vi "Read FieldWidthY.vi"(0 "Field in":refnum<class "Field.lvclass">, 1 "error in (no error)":errorcluster) -> (2 "Field out":refnum<class "Field.lvclass">, 3 "FieldWidthY":i32=55, 4 "error out":errorcluster)   [LabVIEW 2014, in "Field.lvclass"]
uses:
  Field.lvclass
  Field.lvclass/Field.ctl
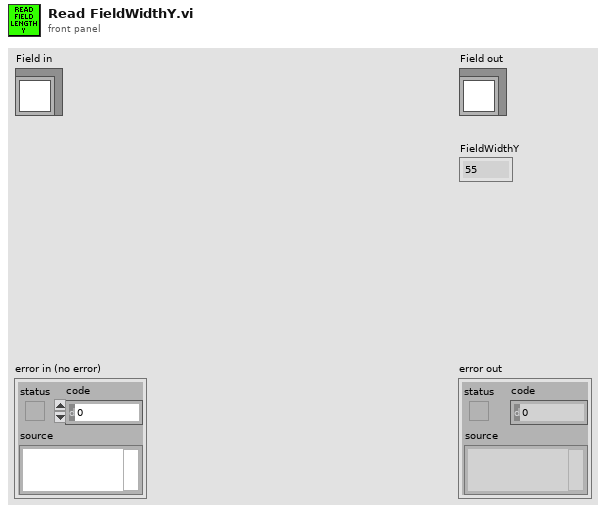
[diagram p1: front panel]
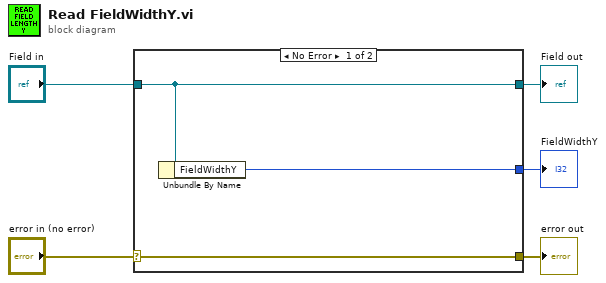
[diagram p0: block diagram]
diagram:
  n1 = case shown="No Error" "error in (no error)" {
    selector: "error in (no error)" -> [w8 w9]
    tunnel: [w8 w9] -> w4
    tunnel: [w7 w10] -> w2
    tunnel: "Field in" -> [w7 w10]
    tunnel: [w6 _] -> w1
    frame No Error {
      n2 = Unbundle By Name(w7) -> ("FieldWidthY"=w6:i32)
    }
    frame Error {
    }
  }
  "error out" <- w4
  "Field out" <- w2
  "FieldWidthY" <- w1
